vi "RX main.vi"   [LabVIEW 2014]
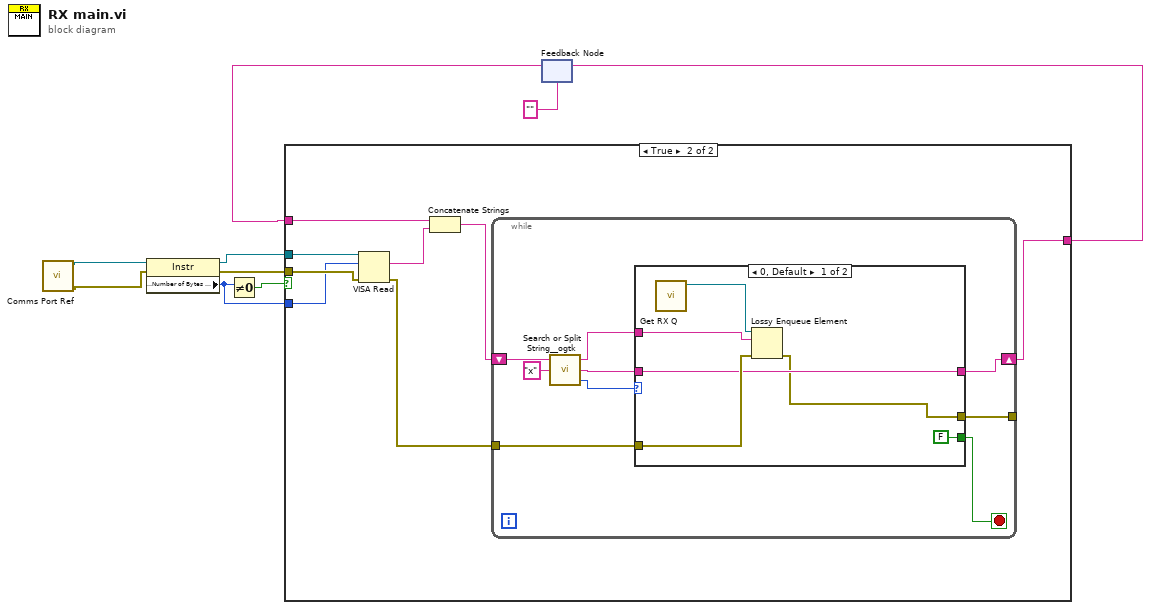
[diagram p0: block diagram]
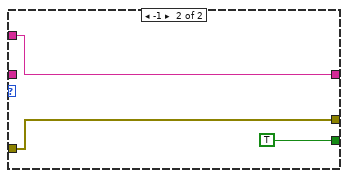
[diagram p3: hidden frame]
diagram:
  n1 = call "Comms Port Ref.vi"() -> ("error out"=w1:errorcluster, "Comms Port Ref"=w2:refnum<visa-resource-name>)  [unwired: 10 in]
  n2 = property class="Instr"(reference=w2, error in=w1) -> (reference out=w8:refnum<visa-resource-name>, error out=w7:errorcluster, "Serial Settings:Number of Bytes at Serial Port"=w3:u32)
  n3 = Not Equal To 0?(x=w3) -> (x != 0?=w9:bool)
  n4 = feedback #1("" ("format string")) -> (w5:string)
  n5 = case shown="True" w9 {
    tunnel: w8 -> [_ w18]
    tunnel: w7 -> [_ w17]
    tunnel: w5 -> [w10 w15]
    tunnel: [w10 w11] -> w4
    tunnel: w3 -> [_ w16]
    frame False {
    }
    frame True {
      n6 = VISA Read(VISA resource name=w18, byte count=w16, error in (no error)=w17) -> (read buffer=w14:string, error out=w12:errorcluster)  [unwired: 2 out]
      n7 = Concatenate Strings(w15, w14) -> (w13:string)
      n8 = while {
        shift-right: [w22] -> w11
        shift-left: w13 -> [w27]
        tunnel: w12 -> [w23]
        tunnel: [w21] -> _
        stop <- w20 stop-if-true
        n9 = call <userlib>:"Search or Split String__ogtk.vi"("search string/char (-)"="x", "string"=w27) -> ("offset after match"=w26:i32, "substring after match"=w24:string, "substring before match"=w25:string)  [unwired: 1 in]
        n10 = case shown="0, Default" w26 {
          tunnel: w25 -> [w28 w36]
          tunnel: w24 -> [w32 _]
          tunnel: w23 -> [w33 w34]
          tunnel: [w32 w36] -> w22
          tunnel: [FALSE TRUE] -> w20
          tunnel: [w30 w34] -> w21
          frame 0, Default {
            n11 = call "Get RX Q.vi"() -> ("RX Q"=w29:refnum<queue>)  [unwired: 10 in, 1 out]
            n12 = Lossy Enqueue Element(queue=w29, element=w28, error in (no error)=w33) -> (error out=w30:errorcluster)  [unwired: 3 out]
          }
          frame -1 {
          }
        }
      }
    }
  }
  n13 = feedback-in #1(w4) -> ()
